vi "Leap Motion - Flex Ext shape data.vi"(8 "Error In":errorcluster, 10 "Event In":string) -> (0 "Error Out":errorcluster, 2 "Flexext cluster":T1)   [LabVIEW 2014]
uses:
  Typedef/flexext_data.ctl
panel:
  in  "Flexext data":T1
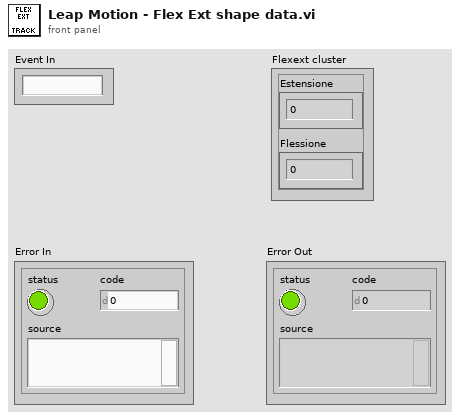
[diagram p1: front panel]
types:
  T1 = typedef "flexext_data.ctl" = cluster{"Estensione":u8, "Flessione":u8}
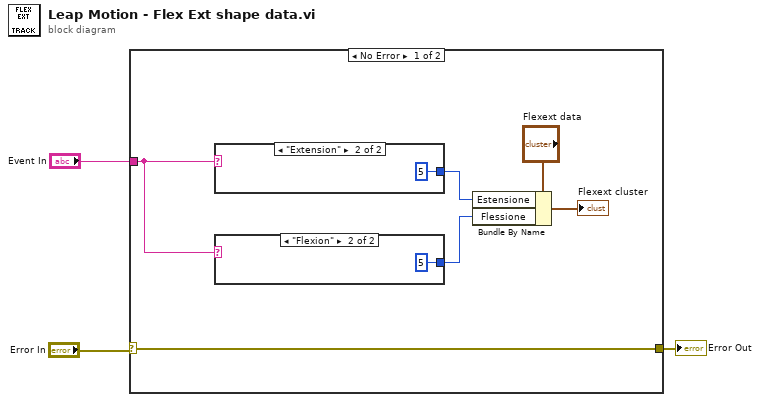
[diagram p0: block diagram]
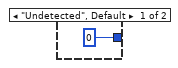
[diagram p2: hidden frame]
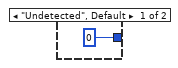
[diagram p3: hidden frame]
diagram:
  n1 = case shown="No Error" "Error In" {
    selector: "Error In" -> [w8 w14]
    tunnel: "Event In" -> [w9 _]
    tunnel: [w8 w14] -> w1
    frame No Error {
      n2 = case shown="\"Extension\"" w9 {
        tunnel: [0 5] -> w6
        frame "Undetected", Default {
        }
        frame "Extension" {
        }
      }
      n3 = case shown="\"Flexion\"" w9 {
        tunnel: [0 5] -> w5
        frame "Undetected", Default {
        }
        frame "Flexion" {
        }
      }
      n4 = Bundle By Name(cluster="Flexext data", "Estensione"=w6, "Flessione"=w5) -> (→"Flexext cluster":T1)
    }
    frame Error {
    }
  }
  "Error Out" <- w1
